vi "Patch_multipart_new.vi"(7 "Headers":string, 8 "error in":errorcluster, 9 "Multpart/Form-Data":T1(array[cluster]), 11 "URL":string) -> (0 "error out":errorcluster, 3 "Multipart PATCH Request":string)   [LabVIEW 2016]
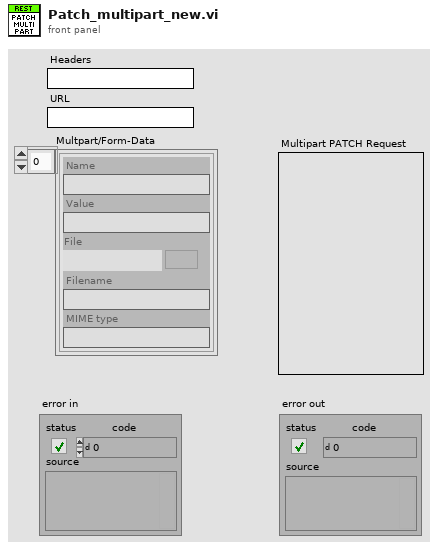
[diagram p1: front panel]
types:
  T1 = cluster{"Name":string, "Value":string, "File":path, "Filename":string, "MIME type":string}[]
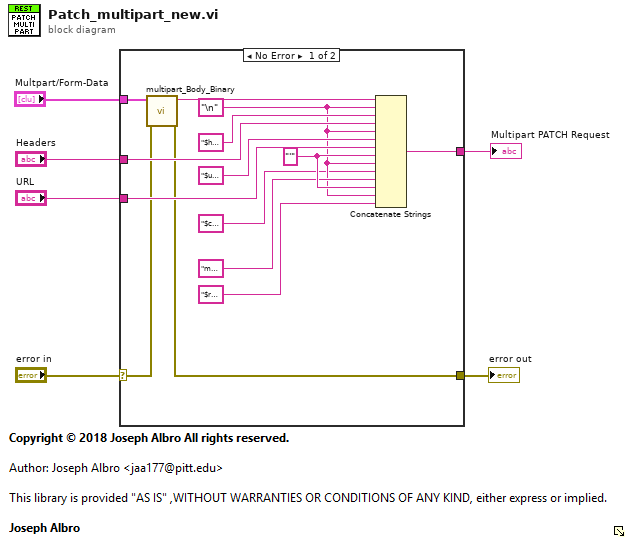
[diagram p0: block diagram]
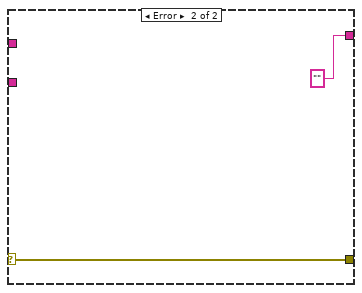
[diagram p2: hidden frame]
diagram:
  n1 = case shown="No Error" "error in" {
    selector: "error in" -> [w8 w21]
    tunnel: "Headers" -> [w20 _]
    tunnel: "URL" -> [w17 _]
    tunnel: [w16 ""] -> w4
    tunnel: [w7 w21] -> w2
    tunnel: "Multpart/Form-Data" -> [w9 _]
    frame No Error {
      w15 = "'" ("string")
      w11 = "\n"
      n2 = call "multipart_Body_Binary.vi"("error in"=w8, "Multpart/Form-Data"=w9) -> ("error out"=w7:errorcluster, "Multipart Binary Body"=w13:string)  [unwired: 8 in]
      n3 = Concatenate Strings(w13, w11, "$headers = ", w20, w11, "$url = '" ("string"), w17, w15, w11, "$contenttype = '" ("string"), "multipart/form-data; boundary=BlockBoundary", w15, w11, "$request = Invoke-WebRequest -Method 'PATCH' -Uri $url -Headers $headers -ContentType $contenttype -InFile 'RequestBodySavedToFile' \nRemove-Item RequestBodySavedToFile" ("string")) -> (w16:string)
    }
    frame Error {
    }
  }
  "Multipart PATCH Request" <- w4
  "error out" <- w2
